vi "bateria.vi"(5 "Characteristic UUID":string, 6 "Connection Status":T1={"MAC Address"="", "cnx handle"=0, "cnx flags"=0, "Address Type"=125, "Connection Interval (ms)"=125, "Timeout(ms)"=125, "Latency"=0, "bonding handle"=0} {"Address Type" items=["Public", "Random"]}, 7 "Service UUID":string, 8 "error in (no error)":errorcluster, 10 "Handle table":string[][](array[string]), 11 "COM Bluegiga in":refnum<visa-resource-name>) -> (0 "error out":errorcluster, 1 "Bateria":string caption="Result", 2 "Numeric":u8, 3 "COM Bluegiga out":refnum<visa-resource-name>)   [LabVIEW 2020]
uses:
  <vilib>/BLE/type_def/connection_status_bundle.ctl
  <vilib>/BLE/type_def/address_type.ctl
panel:
  out "characteristic value":u8[](array[numeric])
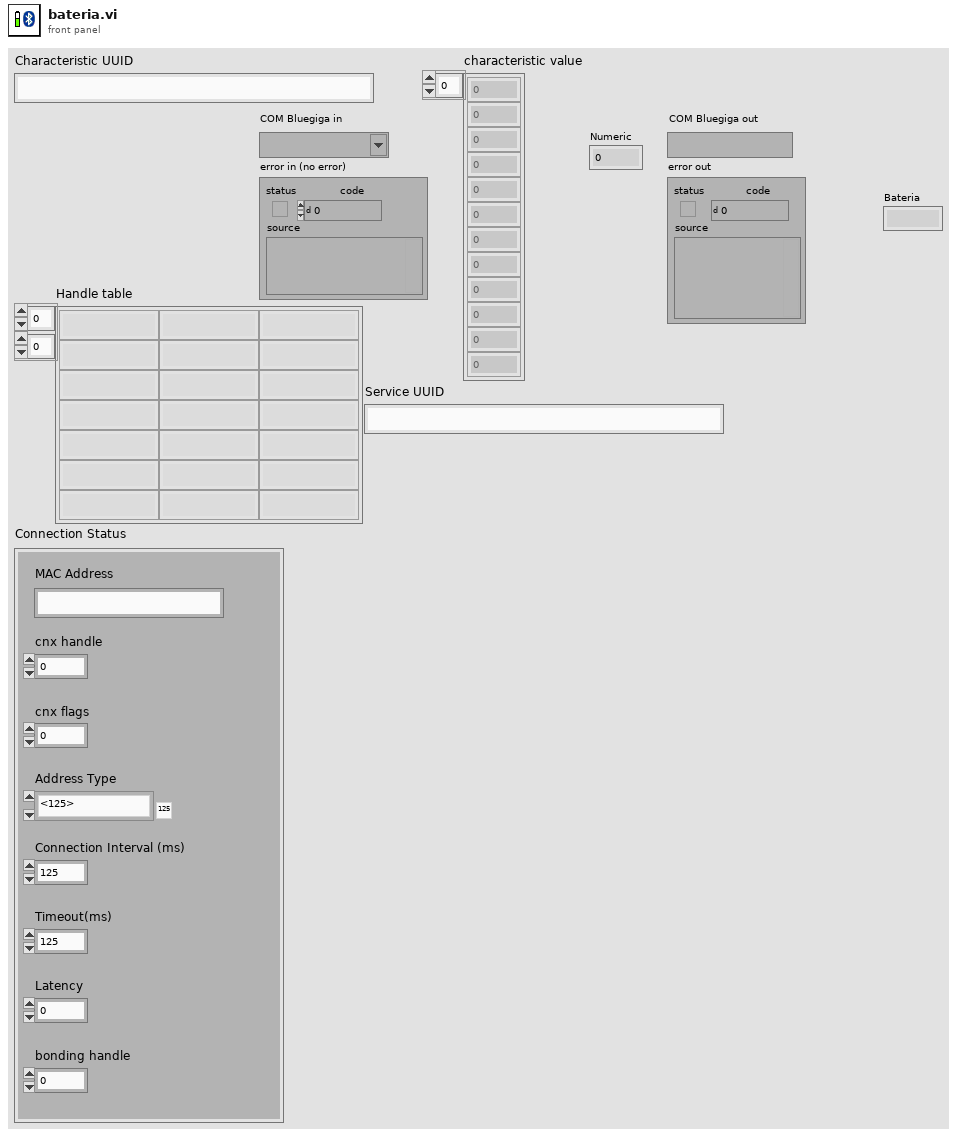
[diagram p1: front panel]
types:
  T1 = typedef "connection_status_bundle.ctl" = cluster{"MAC Address":string, "cnx handle":u8, "cnx flags":u8, "Address Type":T2, "Connection Interval (ms)":u16, "Timeout(ms)":u16, "Latency":u16, "bonding handle":u8}
  T2 = typedef "address_type.ctl" = u8
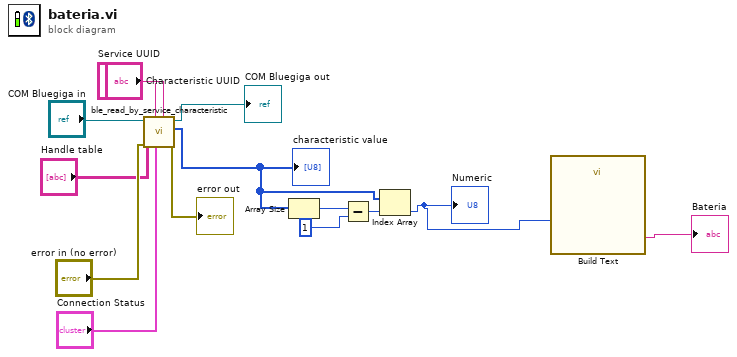
[diagram p0: block diagram]
diagram:
  n1 = call <vilib>:"ble_read_by_service_characteristic.vi"("Characteristic UUID"="Characteristic UUID", "Connection Status"="Connection Status", "Service UUID"="Service UUID", "error in (no error)"="error in (no error)", "Handle table"="Handle table", "COM Bluegiga in"="COM Bluegiga in") -> ("error out"=→"error out":errorcluster, "characteristic value"=w3:u8[], "COM Bluegiga out"=→"COM Bluegiga out":refnum<visa-resource-name>)  [unwired: 3 in]
  "characteristic value" <- w3
  n2 = Array Size(array=w3) -> (size(s)=w12:i32)
  n3 = Subtract(x=w12, y=1) -> (x-y=w14:i32)
  n4 = Index Array(array=w3, index=w14) -> (element=w2:u8)
  "Numeric" <- w2
  n5 = call "Build Text"("B"=w2) -> ("Result"=→"Bateria":string)  [unwired: 13 in, 1 out]
